vi "Initialize.vi"(8 "error in":errorcluster, 11 "Shared Resources in":refnum<class "Shared Resources.lvclass">) -> (0 "error out":errorcluster, 3 "Shared Resources out":refnum<class "Shared Resources.lvclass">)   [LabVIEW 2020, in "AIM MIL-STD-1553 Engine.lvlib" / "Implementation.lvlib" / "Shared Resources.lvclass"]
uses:
  Shared Resources.lvclass
  Shared Resources.lvclass/Shared Resources.ctl
  Custom Device/Custom Device.lvlib
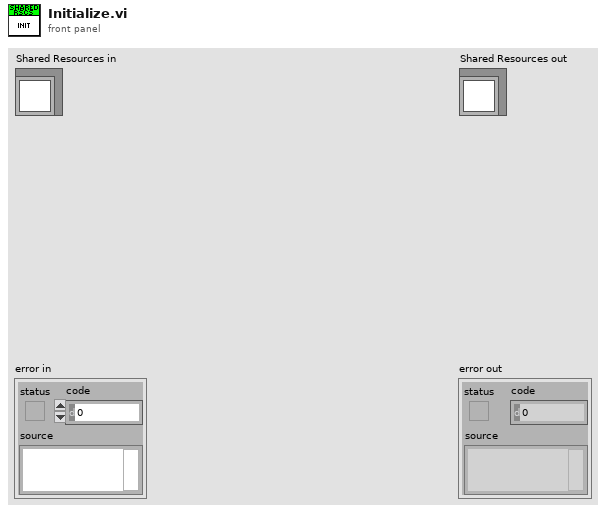
[diagram p1: front panel]
types:
  T1 = typedef "Device Parameters.ctl" = cluster{"initialization method":T2, "card number":i32, "PXI slot number":i32, "core number":i32}
  T2 = typedef "Initialization Method.ctl" = enum16{"PXI Slot Number", "Card Number"}
  T3 = typedef "AIM MIL-STD-1553 Engine.lvlib/Custom Device.lvlib/Logging Configuration.ctl" = cluster{"configured":bool, "directory":string, "file name":string, "timestamp file name":bool, "data word format":T4}
  T4 = typedef "Data Word Format.ctl" = string
  T5 = typedef "AIM MIL-STD-1553 Engine.lvlib/Custom Device.lvlib/Hardware Handles.ctl" = cluster{"core handle":u64, "core reader handle":u64, "channel handles":u64[]}
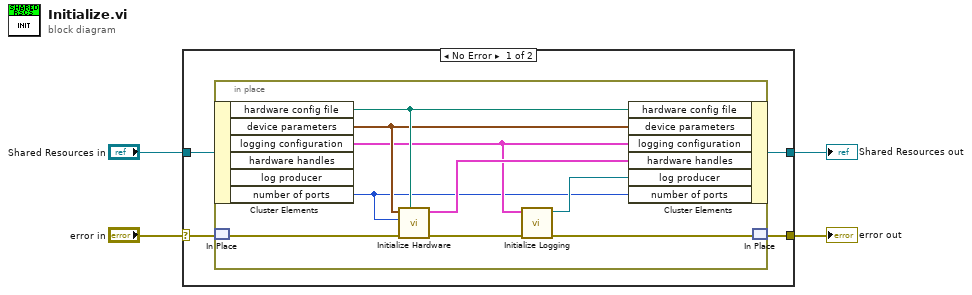
[diagram p0: block diagram]
diagram:
  n1 = case shown="No Error" "error in" {
    selector: "error in" -> [w8 w19]
    tunnel: [w7 w19] -> w1
    tunnel: "Shared Resources in" -> [w6 w18]
    tunnel: [w5 w18] -> w2
    frame No Error {
      n2 = in-place {
        n3 = in-place-cluster #1(w6) -> ("hardware config file"=w16:path, "device parameters"=w15:T1, "logging configuration"=w13:T3, "number of ports"=w9:i32)  [unwired: 2 out]
        n4 = in-place-match #2(w8) -> (w10:errorcluster)
        n5 = call "Initialize Hardware.vi"("hardware config file"=w16, "error in"=w10, "number of ports"=w9, "device parameters"=w15) -> ("error out"=w11:errorcluster, "hardware handles"=w17:T5)  [unwired: 6 in]
        n6 = call "Initialize Logging.vi"("error in"=w11, "logging configuration"=w13) -> ("error out"=w14:errorcluster, "Producer"=w12:refnum<class "Log Producer.lvclass">)  [unwired: 8 in]
        n7 = in-place-cluster #1("hardware config file"=w16, "device parameters"=w15, "logging configuration"=w13, "hardware handles"=w17, "log producer"=w12, "number of ports"=w9) -> (w5:refnum<class "Shared Resources.lvclass">)
        n8 = in-place-match #2(w14) -> (w7:errorcluster)
      }
    }
    frame Error {
    }
  }
  "error out" <- w1
  "Shared Resources out" <- w2
